vi "Mem_WaveformArray.vi"(8 "error in (no error)":errorcluster, 11 "dataInfo":T1) -> (0 "error out":errorcluster, 2 "Array":waveform(dbl)[](array[waveform]))   [LabVIEW 2019, in "Memory Data Access.lvlib"]
uses:
  Memory Data Access.lvlib
  Typedef/memoryDataBlock.ctl
  Global/Global.vi
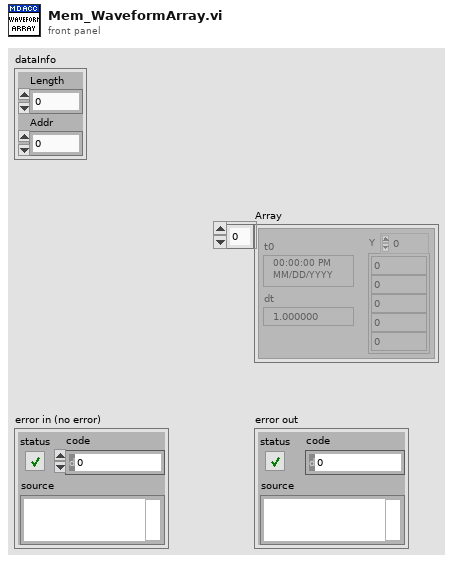
[diagram p1: front panel]
types:
  T1 = typedef "Memory Data Access.lvlib/memoryDataBlock.ctl" = cluster{"Length":u32, "Addr":u64}
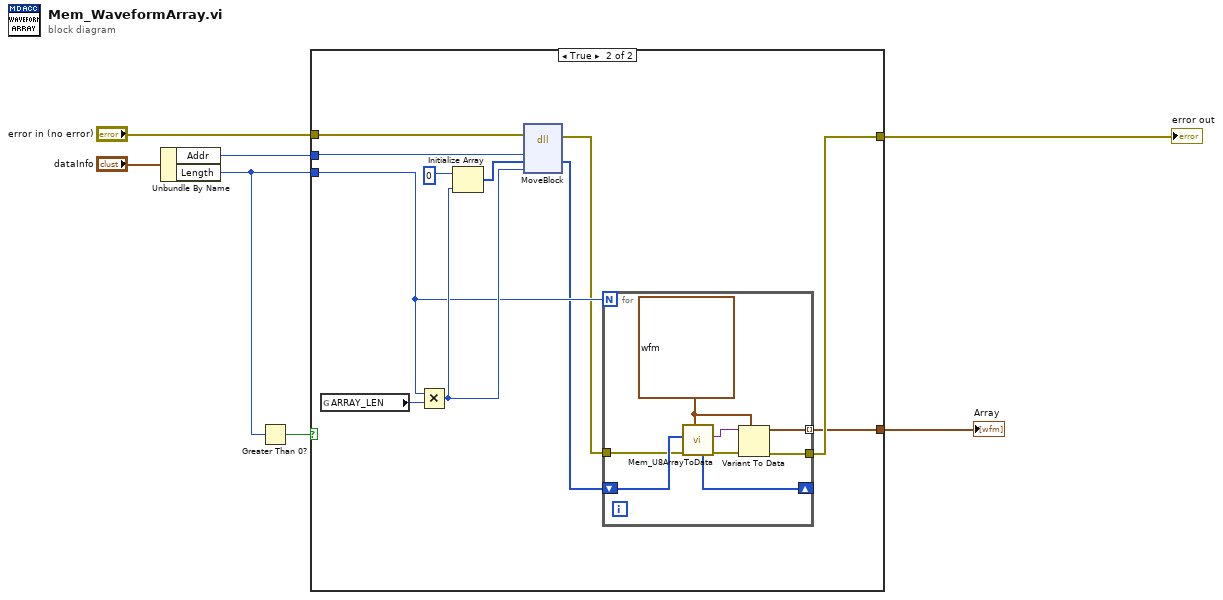
[diagram p0: block diagram]
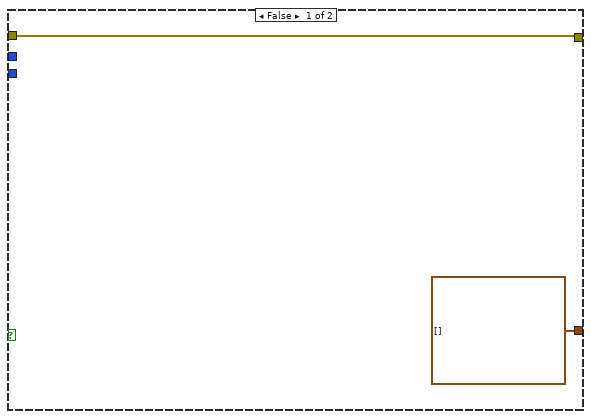
[diagram p2: hidden frame]
diagram:
  n1 = Unbundle By Name("dataInfo") -> ("Addr"=w3:u64, "Length"=w2:u32)
  n2 = Greater Than 0?(x=w2) -> (x > 0?=w5:bool)
  n3 = case shown="True" w5 {
    tunnel: "error in (no error)" -> [w9 w20]
    tunnel: [w9 w11] -> w6
    tunnel: w3 -> [_ w17]
    tunnel: w2 -> [_ w14]
    tunnel: [waveform(dbl)[] [] w10] -> w1
    frame False {
    }
    frame True {
      n4 = global read "Global.vi" "ARRAY_LEN"() -> (w16:u32)
      n5 = Multiply(x=w14, y=w16) -> (x*y=w15:u32)
      n6 = Initialize Array(u8 0, w15) -> (w18:u8[])
      n7 = dll-call lib="LabVIEW" fn="MoveBlock"(error in=w20, "Address"=w17, "Destination"=w18, "Size"=w15) -> (error out=w12:errorcluster, "Destination"=w13:u8[])  [unwired: 5 in, 1 out]
      n8 = for {
        N: w14 -> [_]
        shift-right: [w27] -> _
        shift-left: w13 -> [w28]
        tunnel: [w23] -> w10 mode=indexing
        tunnel: [w22] -> w11
        tunnel: w12 -> [w21]
        w24 = waveform(dbl) {"t0"=timestamp(0 s since 1904-01-01), "dt"=1.0, "Y"=[]} ("Waveform")
        n9 = call "Mem_U8ArrayToData.vi"("Type"=w24, "error in (no error)"=w21, "ByteArray"=w28) -> ("error out"=w26:errorcluster, "data"=w25:variant, "ByteArray Left"=w27:u8[])  [unwired: 5 in, 1 out]
        n10 = Variant To Data(error in=w26, type=w24, Variant=w25) -> (data=w23:waveform(dbl), error out=w22:errorcluster)
      }
    }
  }
  "error out" <- w6
  "Array" <- w1
